vi "Test Assert Greater Or Equal.vi"(8 "error in (no error)":errorcluster) -> (0 "error out":errorcluster)   [LabVIEW 2013]
uses:
  classes/Assert/Assert.lvclass
  classes/Test/Test.lvclass
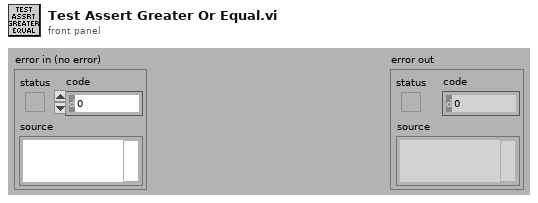
[diagram p1: front panel]
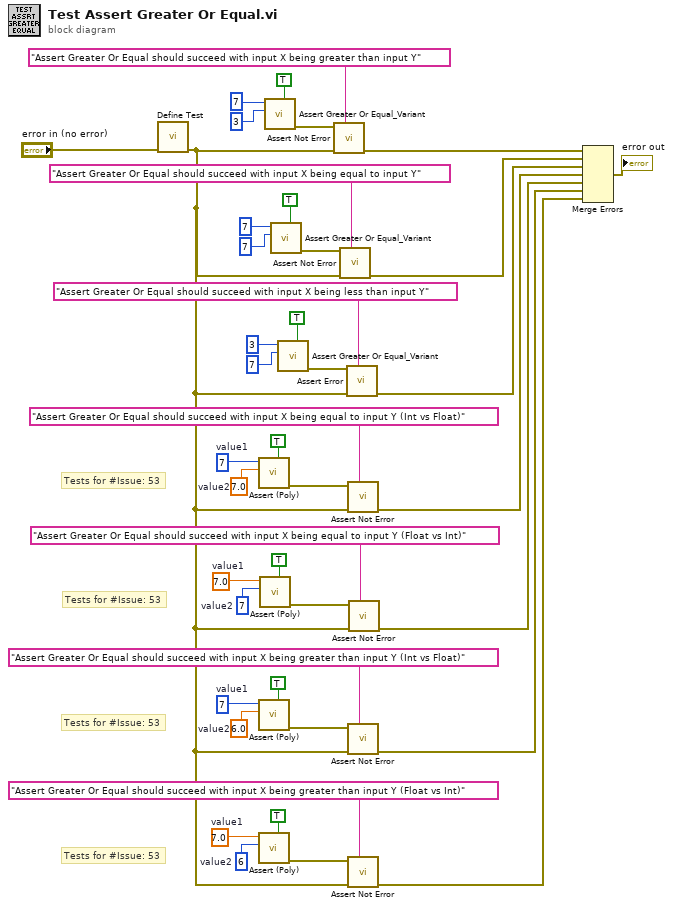
[diagram p0: block diagram]
diagram:
  w3 = 6  # value2
  w4 = 7.0  # value1
  w13 = 7  # value2
  w12 = 7.0  # value1
  w19 = 6.0  # value2
  w18 = 7  # value1
  w20 = 7.0  # value2
  w21 = 7  # value1
  # "Tests for #Issue: 53"
  # "Tests for #Issue: 53"
  # "Tests for #Issue: 53"
  # "Tests for #Issue: 53"
  n1 = call "Define Test.vi"("error in (no error)"="error in (no error)") -> ("error out"=w2:errorcluster)  [unwired: 10 in]
  n2 = call-poly "Assert (Poly).vi"("Assert Only? (F)"=TRUE, "Y"=w20, "X"=w21) -> ("error out"=w23:errorcluster)  [unwired: 8 in]
  n3 = call-poly "Assert (Poly).vi"("Assert Only? (F)"=TRUE, "Y"=w19, "X"=w18) -> ("error out"=w16:errorcluster)  [unwired: 8 in]
  n4 = call-poly "Assert (Poly).vi"("Assert Only? (F)"=TRUE, "Y"=w3, "X"=w4) -> ("error out"=w6:errorcluster)  [unwired: 8 in]
  n5 = call-poly "Assert (Poly).vi"("Assert Only? (F)"=TRUE, "Y"=w13, "X"=w12) -> ("error out"=w10:errorcluster)  [unwired: 8 in]
  n6 = call "Assert Greater Or Equal_Variant.vi"("Assert Only? (F)"=TRUE, "Y"=3, "X"=7) -> ("error out"=w45:errorcluster)  [unwired: 8 in]
  n7 = call "Assert Greater Or Equal_Variant.vi"("Assert Only? (F)"=TRUE, "Y"=7, "X"=7) -> ("error out"=w43:errorcluster)  [unwired: 8 in]
  n8 = call "Assert Greater Or Equal_Variant.vi"("Assert Only? (F)"=TRUE, "Y"=7, "X"=3) -> ("error out"=w31:errorcluster)  [unwired: 8 in]
  n9 = call "Assert Not Error.vi"("Label"="Assert Greater Or Equal should succeed with input X being greater than input Y", "error in (no error)"=w2, "Not Error?"=w45) -> ("error out"=w37:errorcluster)  [unwired: 8 in]
  n10 = call "Assert Not Error.vi"("Label"="Assert Greater Or Equal should succeed with input X being equal to input Y", "error in (no error)"=w2, "Not Error?"=w43) -> ("error out"=w38:errorcluster)  [unwired: 8 in]
  n11 = call "Assert Error.vi"("Label"="Assert Greater Or Equal should succeed with input X being less than input Y", "error in (no error)"=w2, "Error?"=w31) -> ("error out"=w26:errorcluster)  [unwired: 8 in]
  n12 = call "Assert Not Error.vi"("Label"="Assert Greater Or Equal should succeed with input X being equal to input Y (Int vs Float)", "error in (no error)"=w2, "Not Error?"=w23) -> ("error out"=w24:errorcluster)  [unwired: 8 in]
  n13 = call "Assert Not Error.vi"("Label"="Assert Greater Or Equal should succeed with input X being greater than input Y (Int vs Float)", "error in (no error)"=w2, "Not Error?"=w16) -> ("error out"=w14:errorcluster)  [unwired: 8 in]
  n14 = call "Assert Not Error.vi"("Label"="Assert Greater Or Equal should succeed with input X being greater than input Y (Float vs Int)", "error in (no error)"=w2, "Not Error?"=w6) -> ("error out"=w1:errorcluster)  [unwired: 8 in]
  n15 = call "Assert Not Error.vi"("Label"="Assert Greater Or Equal should succeed with input X being equal to input Y (Float vs Int)", "error in (no error)"=w2, "Not Error?"=w10) -> ("error out"=w8:errorcluster)  [unwired: 8 in]
  n16 = Merge Errors(w37, w38, w26, w24, w8, w14, w1) -> (→"error out":errorcluster)
